vi "SeCrTS-DD NS Data Storage.vi"(7 "NOT DIS Out":T1, 8 "error in":errorcluster, 9 "AI_V_Data P\nAI_C_Data P\nAO_Data P\nDO_Data P\nACC_Data P\nTC Data P\nDrive_A_C \nDrive_A_D\nAI_C_Data S\nDO_Data S":refnum<queue>[](array[refnum]), 10 "Data in":string, 11 "DI P\nDI S":refnum<queue>[](array[refnum])) -> (0 "error out":errorcluster)   [LabVIEW 2022 SP3]
uses:
  Control/SeCrTS-Notifier Ref.ctl
panel:
  out "overflow? 5":bool
  out "overflow? 3":bool
  out "overflow? 2":bool
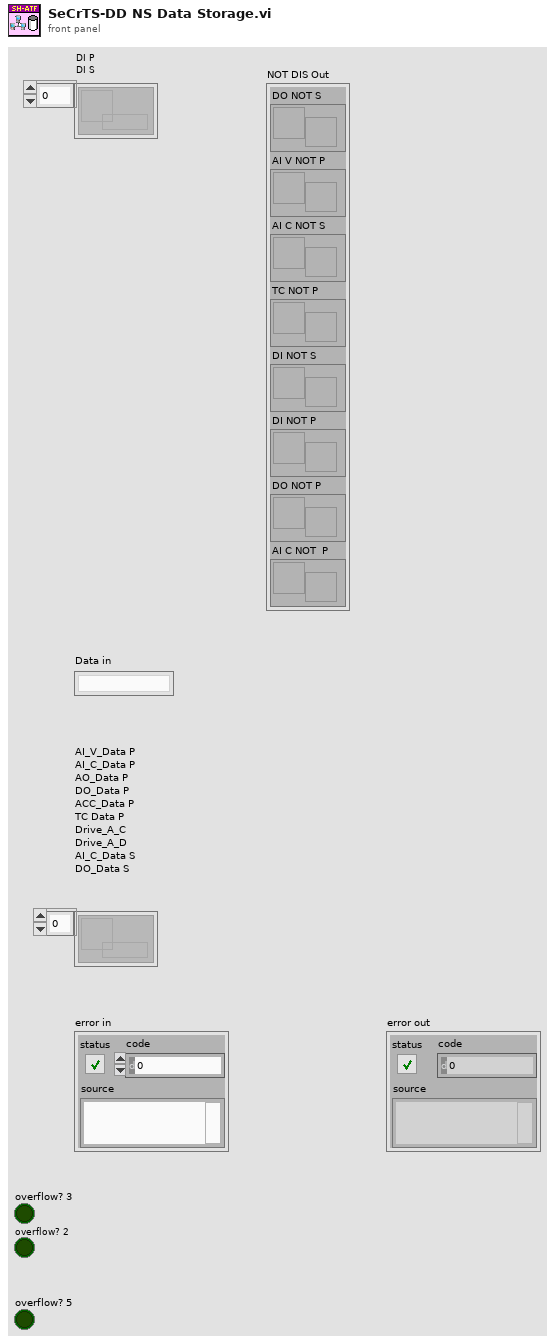
[diagram p1: front panel]
types:
  T1 = typedef "SeCrTS-Notifier Ref.ctl" = cluster{"DO NOT S":refnum<notifier>, "AI V NOT P":refnum<notifier>, "AI C NOT S":refnum<notifier>, "TC NOT P":refnum<notifier>, "DI NOT S":refnum<notifier>, "DI NOT P":refnum<notifier>, "DO NOT P":refnum<notifier>, "AI C NOT  P":refnum<notifier>}
  T2 = cluster{"AI_V_Data":waveform(dbl)[][], "AI_C_Data":waveform(dbl)[][], "AO_Data":waveform(dbl)[][], "DO_Data":waveform(dbl)[][], "DI_Data":digitalwaveform[][], "ACC_Data":waveform(dbl)[][], "TC Data":waveform(dbl)[][], "Drive_A_C":waveform(dbl)[][], "Drive_A_D":waveform(dbl)[][], "Drive_L_C":waveform(dbl)[][], "Drive_L_D":waveform(dbl)[][]}
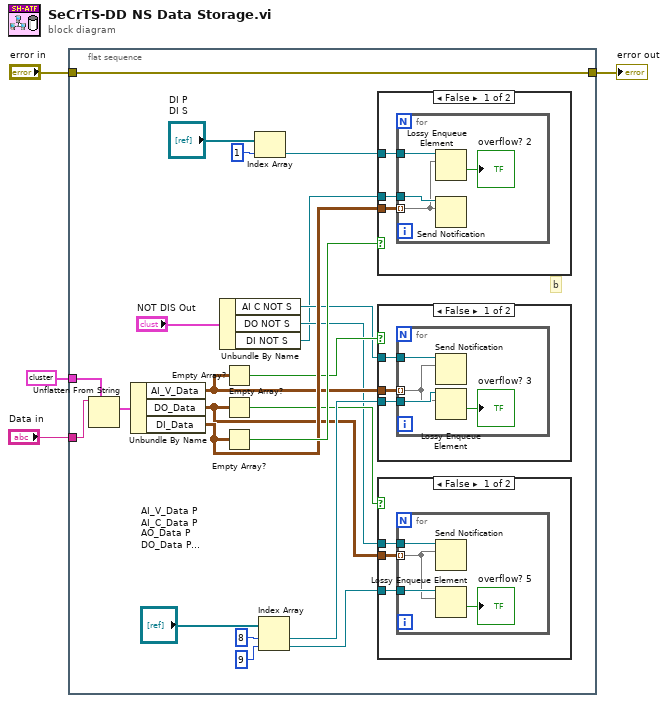
[diagram p0: block diagram]
diagram:
  n1 = flat-sequence {
    tunnel: T2 data[101848B] ("data out") -> [w8]
    tunnel: "Data in" -> [w7]
    tunnel: "error in" -> [w5]
    tunnel: [w5] -> w1
    frame #0 {
      # "b"
      n2 = Unflatten From String(type=w8, binary string=w7) -> (value=w6:T2)  [unwired: 3 in, 2 out]
      n3 = Unbundle By Name(w6) -> ("AI_V_Data"=w20:waveform(dbl)[][], "DO_Data"=w18:waveform(dbl)[][], "DI_Data"=w22:digitalwaveform[][])
      n4 = Unbundle By Name("NOT DIS Out") -> ("AI C NOT S"=w17:refnum<notifier>, "DO NOT S"=w16:refnum<notifier>, "DI NOT S"=w15:refnum<notifier>)
      n5 = Empty Array?(array=w20) -> (empty?=w21:bool)
      n6 = Empty Array?(array=w18) -> (empty?=w19:bool)
      n7 = Empty Array?(array=w22) -> (empty?=w23:bool)
      n8 = Index Array(array="DI P\nDI S", index=1) -> (element=w10:refnum<queue>)
      n9 = Index Array(array="AI_V_Data P\nAI_C_Data P\nAO_Data P\nDO_Data P\nACC_Data P\nTC Data P\nDrive_A_C \nDrive_A_D\nAI_C_Data S\nDO_Data S", index #1=8 ("index"), index #2=9 ("index")) -> (element #1=w25:refnum<queue>, element #2=w12:refnum<queue>)
      n10 = case shown="False" w23 {
        tunnel: w22 -> [w43 _]
        tunnel: w10 -> [w42 _]
        tunnel: w15 -> [w41 _]
        frame False {
          n11 = for {
            tunnel: w43 -> [w44] mode=indexing
            tunnel: w42 -> [w47]
            tunnel: w41 -> [w45]
            n12 = Lossy Enqueue Element(queue=w47, element=w44) -> (overflow?=→"overflow? 2":bool)  [unwired: 1 in, 3 out]
            n13 = Send Notification(notification=w44, notifier=w45) -> ()  [unwired: 1 in, 2 out]
          }
        }
        frame True {
        }
      }
      n14 = case shown="False" w21 {
        tunnel: w20 -> [w36 _]
        tunnel: w25 -> [w35 _]
        tunnel: w17 -> [w34 _]
        frame False {
          n15 = for {
            tunnel: w36 -> [w37] mode=indexing
            tunnel: w35 -> [w40]
            tunnel: w34 -> [w38]
            n16 = Send Notification(notification=w37, notifier=w38) -> ()  [unwired: 1 in, 2 out]
            n17 = Lossy Enqueue Element(queue=w40, element=w37) -> (overflow?=→"overflow? 3":bool)  [unwired: 1 in, 3 out]
          }
        }
        frame True {
        }
      }
      n18 = case shown="False" w19 {
        tunnel: w18 -> [w29 _]
        tunnel: w12 -> [w28 _]
        tunnel: w16 -> [w27 _]
        frame False {
          n19 = for {
            tunnel: w29 -> [w30] mode=indexing
            tunnel: w28 -> [w33]
            tunnel: w27 -> [w31]
            n20 = Send Notification(notification=w30, notifier=w31) -> ()  [unwired: 1 in, 2 out]
            n21 = Lossy Enqueue Element(queue=w33, element=w30) -> (overflow?=→"overflow? 5":bool)  [unwired: 1 in, 3 out]
          }
        }
        frame True {
        }
      }
    }
  }
  "error out" <- w1
